vi "camera-write_exposure-time-raw.vi"(6 "error in (no error)":errorcluster, 8 "Numeric":i16, 9 "IMAQ Session In":refnum<k11>) -> (0 "error out":errorcluster, 1 "Data":string, 2 "Address":string, 3 "IMAQ Session Out":refnum<k11>)   [LabVIEW 2012]
panel:
  out "Loop Iteration":i32
  out "ACK/NAK":string
  out "String to Write":string
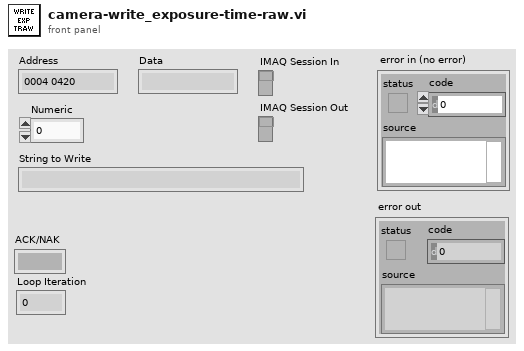
[diagram p1: front panel]
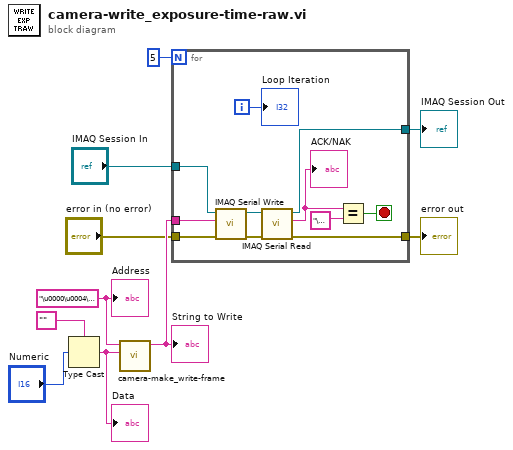
[diagram p0: block diagram]
diagram:
  w10 = "\u0000\u0004\u0004`" ("Address")
  n1 = Type Cast(type="" ("Address"), x="Numeric") -> (*(type *) &x=w1:string)
  "Data" <- w1
  n2 = call "camera-make_write-frame.vi"("Data"=w1, "Address"=w10) -> ("Serial String"=w7:string)  [unwired: 9 in]
  "String to Write" <- w7
  n3 = for {
    N: 5 -> [_]
    tunnel: "IMAQ Session In" -> [w21]
    tunnel: w7 -> [w20]
    tunnel: [w19] -> w6
    tunnel: "error in (no error)" -> [w18]
    tunnel: [w16] -> w4
    i -> [w12]
    stop <- w15 stop-if-true
    n4 = call <vilib>:"IMAQ Serial Write.vi"("error in (no error)"=w18, "String to write"=w20, "IMAQ Session In"=w21) -> ("error out"=w17:errorcluster, "IMAQ Session Out"=w11:refnum<k11>)  [unwired: 5 in]
    n5 = call <vilib>:"IMAQ Serial Read.vi"("error in (no error)"=w17, "IMAQ Session In"=w11) -> ("error out"=w16:errorcluster, "String Read"=w14:string, "IMAQ Session Out"=w19:refnum<k11>)  [unwired: 4 in, 1 out]
    "ACK/NAK" <- w14
    n6 = Equal?(x=w14, y="\u0006") -> (x = y?=w15:bool)
    "Loop Iteration" <- w12
  }
  "IMAQ Session Out" <- w6
  "error out" <- w4
  "Address" <- w10
